vi "WriteBaseActor.vi"(7 "Actor":refnum<class "Actor.lvclass">, 11 "BaseActor":T1) -> (5 "Actor":refnum<class "Actor.lvclass">)   [LabVIEW 2020, in "jettl.lvlib" / "Actor.lvclass"]
uses:
  Actor.lvclass
  Lifetime.ctl
  jettl.lvlib
  Message/Message.lvclass
  MessageSet.ctl
  Messages.ctl
  Message.ctl
  ActorType.ctl
  Actor.ctl
  ComponentActorMap.ctl
  BaseActor.ctl
  TellComponentMap.ctl
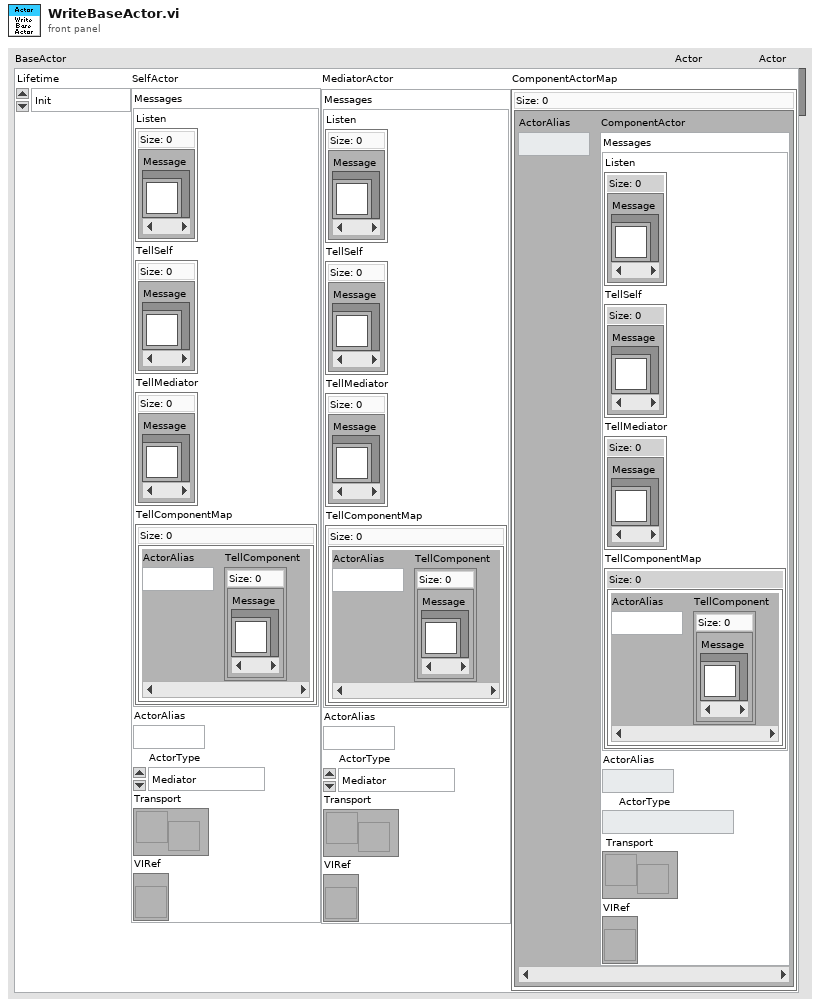
[diagram p1: front panel]
types:
  T1 = typedef "jettl.lvlib/BaseActor.ctl" = cluster{"Lifetime":T2, "SelfActor":T3, "MediatorActor":T3, "ComponentActorMap":T8}
  T2 = typedef "jettl.lvlib/Lifetime.ctl" = enum16{"Init", "Spawn", "Setup", "TeardownBeforeRunning", "Running", "StopCalled", "StoppingWithComponents", "StoppingNoComponents", "TeardownAfterRunning", "Stopped"}
  T3 = typedef "jettl.lvlib/Actor.ctl" = cluster{"Messages":T4, "ActorAlias":string, "ActorType":T7, "Transport":refnum<user-event>, "VIRef":refnum<vi>}
  T4 = typedef "jettl.lvlib/Messages.ctl" = cluster{"Listen":T5, "TellSelf":T5, "TellMediator":T5, "TellComponentMap":T6}
  T5 = typedef "jettl.lvlib/MessageSet.ctl" = set{refnum<class "Message.lvclass">}
  T6 = typedef "jettl.lvlib/TellComponentMap.ctl" = map{string, T5}
  T7 = typedef "jettl.lvlib/ActorType.ctl" = enum16{"Mediator", "Component"}
  T8 = typedef "jettl.lvlib/ComponentActorMap.ctl" = map{string, T3}
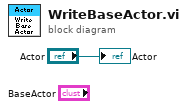
[diagram p0: block diagram]
diagram:
  "Actor" <- "Actor"
